vi "Gate Trigger.vi"(10 "Gate Signal'":bool, 11 "Trigger":bool) -> (3 "Ref Trig":bool)   [LabVIEW 2012]
doc: "This VI gates the Trigger Input based on GateSignal'.\nGate Signal is detected on rising edge and gate is held high until Reference Trigger is detected"
uses:
  <instrlib>/FlexRIO/Libraries/Helper VIs/NI FlexRIO Helper VIs.lvlib
panel:
  # "This VI gates the Trigger Input  based on GateSignal'.\nGate Signal is detected on rising edge and gate is held high until Reference Trigger is detected"
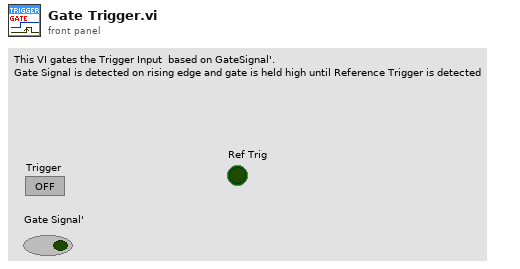
[diagram p1: front panel]
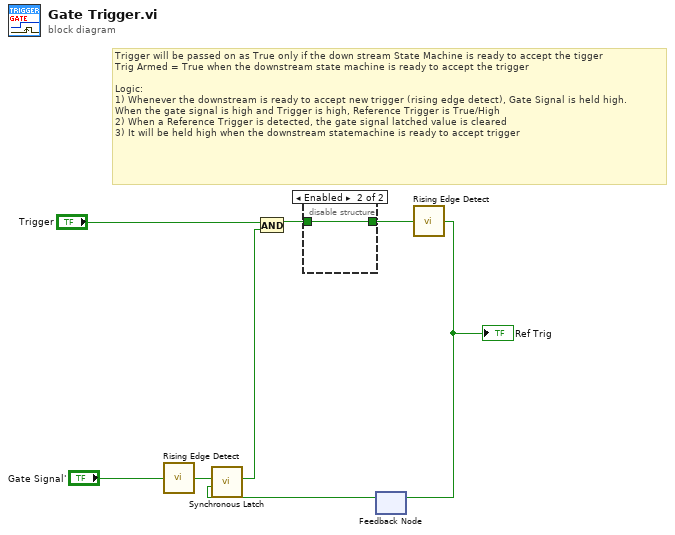
[diagram p0: block diagram]
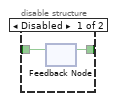
[diagram p2: hidden frame]
diagram:
  # "Trigger will be passed on as True only if the down stream State Machine is ready to accept the tigger\nTrig Armed = True when the downstream state machine is ready to accept the trigger\n\nLogic:\n1) Whenever the downstream is ready to accept new trigger (rising edge detect), Gate Signal is held high.\nWhen the gate signal is high and Trigger is high, Reference Trigger is True/High\n2) When a Reference Trigger is detected, the gate signal latched value is cleared\n3) It will be held high when the downstream statemachine is ready to accept trigger"
  n1 = call <instrlib>:"Rising Edge Detect.vi"("signal"="Gate Signal'") -> ("edge detected"=w7:bool)  [unwired: 14 in]
  n2 = feedback #1() -> (w8:bool)  [unwired: 1 in]
  n3 = call <instrlib>:"Synchronous Latch.vi"("clear"=w8, "set"=w7) -> ("out"=w4:bool)  [unwired: 9 in]
  n4 = And(x="Trigger", y=w4) -> (x .and. y?=w5:bool)
  n5 = disable-structure shown="Enabled" {
    disable-tunnel: w5 -> [w10 w11]
    disable-tunnel: [w9 w11] -> w2
    frame Disabled {
      n6 = feedback #2() -> (w9:bool)  [unwired: 1 in]
      n7 = feedback-in #2(w10) -> ()
    }
    frame Enabled {
    }
  }
  n8 = call <instrlib>:"Rising Edge Detect.vi"("signal"=w2) -> ("edge detected"=w6:bool)  [unwired: 14 in]
  "Ref Trig" <- w6
  n9 = feedback-in #1(w6) -> ()
